vi "write_new_value.vi"(8 "error in (no error)":errorcluster, 9 "Value":variant, 10 "Data Name (Use Value Name)":string, 11 "CurrentValueTable in":refnum<class "CurrentValueTable.lvclass">) -> (0 "error out":errorcluster, 3 "CurrentValueTable out":refnum<class "CurrentValueTable.lvclass">)   [LabVIEW 2015, in "CurrentValueTable.lvlib" / "CurrentValueTable.lvclass"]
uses:
  CurrentValueTable.lvclass
  CurrentValueTable.lvclass/CurrentValueTable.ctl
  <vilib>/Utility/Data Type/NI_Data Type.lvlib
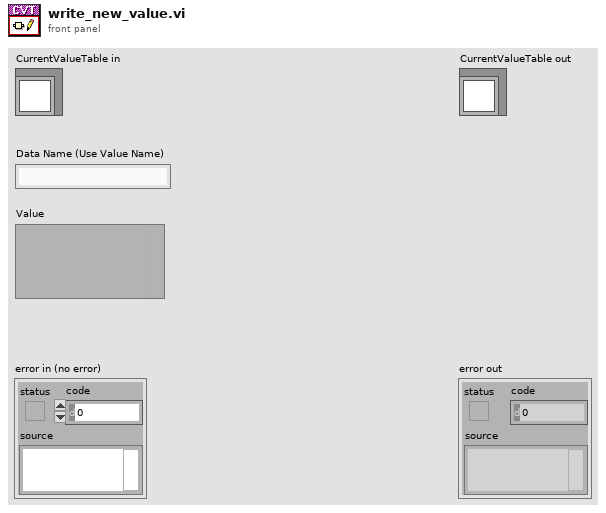
[diagram p1: front panel]
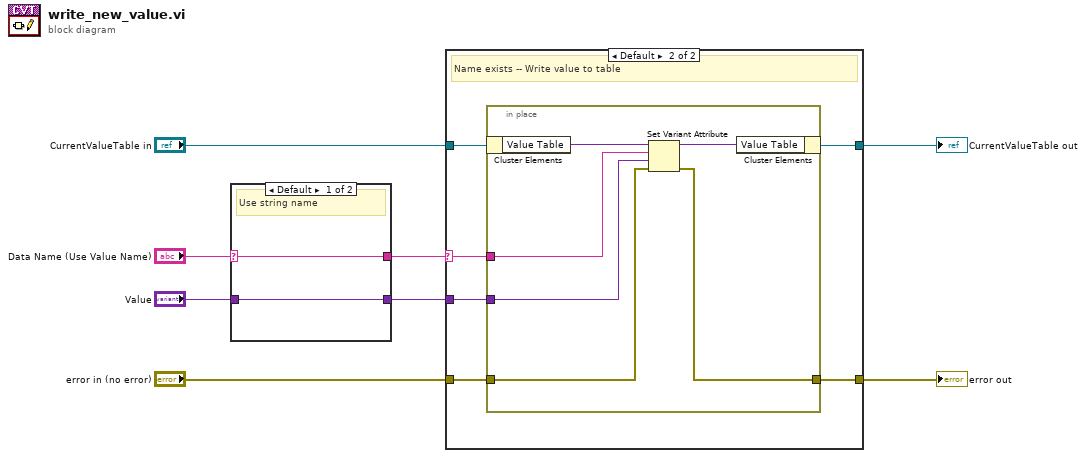
[diagram p0: block diagram]
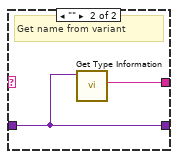
[diagram p2: hidden frame]
diagram:
  n1 = case shown="Default" "Data Name (Use Value Name)" {
    selector: "Data Name (Use Value Name)" -> [w10 _]
    tunnel: "Value" -> [w9 w11]
    tunnel: [w10 w12] -> w1
    tunnel: [w9 w11] -> w2
    frame Default {
      # "Use string name"
    }
    frame "" {
      # "Get name from variant"
      n2 = call <vilib>:"Get Type Information.vi"("Variant"=w11) -> ("Name"=w12:string)  [unwired: 6 in, 4 out]
    }
  }
  n3 = case shown="Default" w1 {
    selector: w1 -> [_ w17]
    tunnel: "CurrentValueTable in" -> [w14 w16]
    tunnel: [w14 w15] -> w7
    tunnel: "error in (no error)" -> [w13 w20]
    tunnel: [w13 w19] -> w5
    tunnel: w2 -> [_ w18]
    frame "" {
      # "No name available -- Skip writing unnamed datum"
    }
    frame Default {
      # "Name exists -- Write value to table"
      n4 = in-place {
        in-place-border: w20 -> [w26]
        in-place-border: [w25] -> w19
        in-place-border: w18 -> [w24]
        in-place-border: w17 -> [w23]
        n5 = in-place-cluster #1(w16) -> ("Value Table"=w22:variant)
        n6 = Set Variant Attribute(Variant=w22, name=w23, value=w24, error in=w26) -> (Variant out=w21:variant, error out=w25:errorcluster)  [unwired: 1 out]
        n7 = in-place-cluster #1("Value Table"=w21) -> (w15:refnum<class "CurrentValueTable.lvclass">)
      }
    }
  }
  "error out" <- w5
  "CurrentValueTable out" <- w7
